vi "create report.vi"(8 "error in (no error)":errorcluster, 11 "TomoConversion in":refnum<class "TomoConversion.lvclass">) -> (0 "error out":errorcluster, 1 "correct number of subfolders":i32, 2 "Array":dbl[][](array[numeric]), 3 "TomoConversion out":refnum<class "TomoConversion.lvclass">)   [LabVIEW 2012, in "TomoConversion.lvclass"]
uses:
  TomoConversion.lvclass
  TomoConversion.lvclass/TomoConversion.ctl
  notice type.ctl
panel:
  out "j number y folders in this x 2":i32
  out "j number y folders in this x":i32
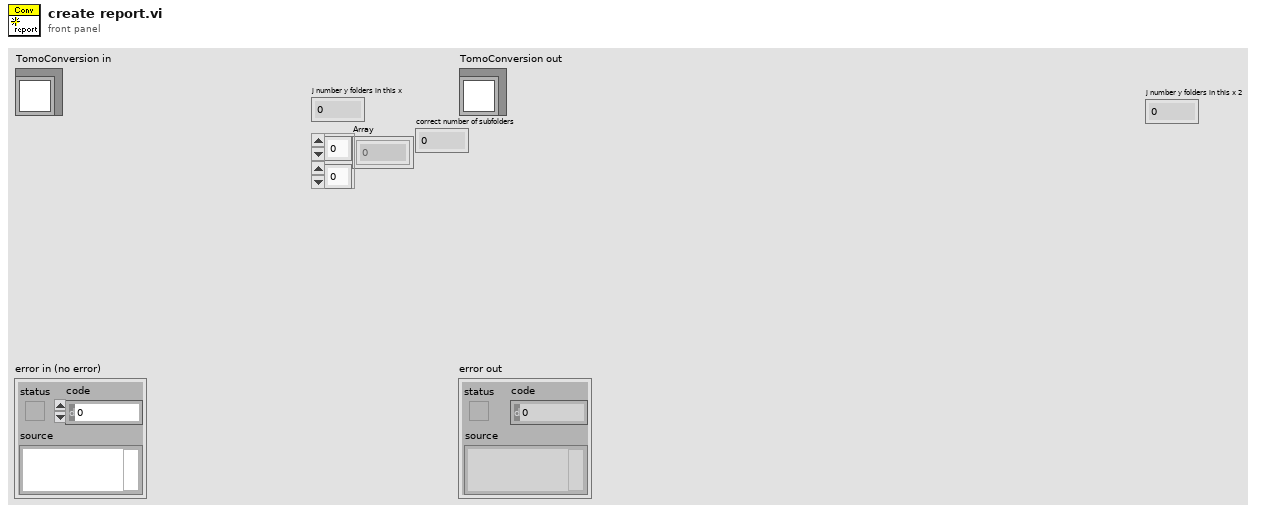
[diagram p1: front panel]
types:
  T1 = typedef "TomoConversion.lvclass/notice type.ctl" = enum16{"Grotto", "folder issue"}
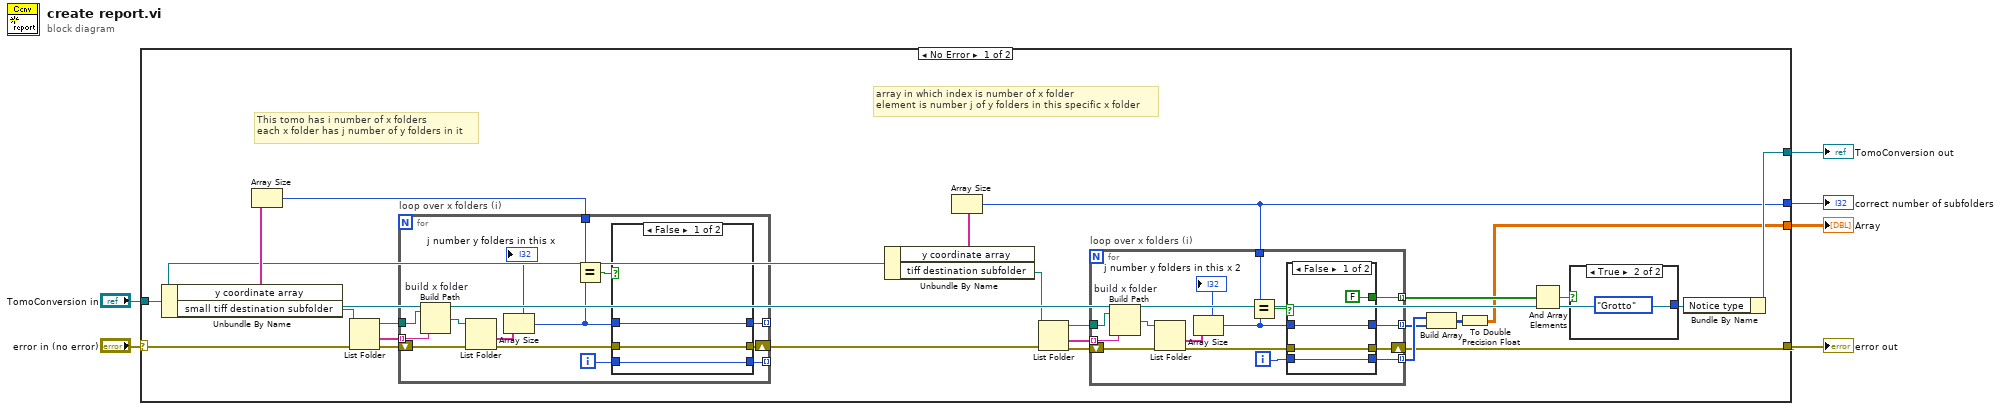
[diagram p0: block diagram]
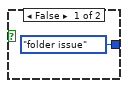
[diagram p2: hidden frame]
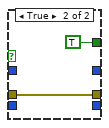
[diagram p3: hidden frame]
diagram:
  n1 = case shown="No Error" "error in (no error)" {
    selector: "error in (no error)" -> [w30 w71]
    tunnel: [w10 w71] -> w5
    tunnel: [w19 w70] -> w3
    tunnel: "TomoConversion in" -> [w20 w70]
    tunnel: [w8 _] -> w2
    tunnel: [w7 _] -> w1
    frame No Error {
      # "array in which index is number of x folder\nelement is number j of y folders in this specific x folder"
      # "This tomo has i number of x folders \neach x folder has j number of y folders in it"
      n2 = Unbundle By Name(w20) -> ("y coordinate array"=w26:string[], "small tiff destination subfolder"=w25:path)
      n3 = Array Size(array=w26) -> (size(s)=w16:i32)
      n4 = List Folder(path=w25, error in=w30) -> (path out=w27:path, folder names=w29:string[], error out=w28:errorcluster)  [unwired: 2 in, 1 out]
      n5 = for "loop over x folders (i)" {
        tunnel: w29 -> [w64] mode=indexing
        tunnel: w27 -> [w65]
        tunnel: [w54] -> _ mode=indexing
        shift-right: [w56] -> w15
        shift-left: w28 -> [w62]
        tunnel: w16 -> [w60]
        tunnel: [w53] -> _ mode=indexing
        i -> [w55]
        n6 = Build Path "build x folder"(base path=w65, name or relative path=w64) -> (appended path=w63:path)
        n7 = List Folder(path=w63, error in=w62) -> (folder names=w61:string[], error out=w57:errorcluster)  [unwired: 2 in, 2 out]
        n8 = Array Size(array=w61) -> (size(s)=w58:i32)
        "j number y folders in this x" <- w58
        n9 = Equal?(x=w60, y=w58) -> (x = y?=w59:bool)
        n10 = case shown="False" w59 {
          tunnel: w58 -> [w67 _]
          tunnel: [w67 _] -> w54
          tunnel: w57 -> [w68 w69]
          tunnel: [w68 w69] -> w56
          tunnel: w55 -> [w66 _]
          tunnel: [w66 _] -> w53
          frame False {
          }
          frame True {
            # "correct number of subfolders"
          }
        }
      }
      n11 = Unbundle By Name(w20) -> ("y coordinate array"=w24:string[], "tiff destination subfolder"=w11:path)
      n12 = Array Size(array=w24) -> (size(s)=w8:i32)
      n13 = List Folder(path=w11, error in=w15) -> (path out=w23:path, folder names=w21:string[], error out=w22:errorcluster)  [unwired: 2 in, 1 out]
      n14 = for "loop over x folders (i)" {
        tunnel: w21 -> [w45] mode=indexing
        tunnel: w23 -> [w46]
        tunnel: [w36] -> w12 mode=indexing
        shift-right: [w37] -> w10
        shift-left: w22 -> [w43]
        tunnel: w8 -> [w41]
        tunnel: [w34] -> w9 mode=indexing
        tunnel: [w33] -> w13 mode=indexing
        i -> [w35]
        n15 = Build Path "build x folder"(base path=w46, name or relative path=w45) -> (appended path=w44:path)
        n16 = List Folder(path=w44, error in=w43) -> (folder names=w42:string[], error out=w40:errorcluster)  [unwired: 2 in, 2 out]
        n17 = Array Size(array=w42) -> (size(s)=w38:i32)
        "j number y folders in this x 2" <- w38
        n18 = Equal?(x=w41, y=w38) -> (x = y?=w39:bool)
        n19 = case shown="False" w39 {
          tunnel: w40 -> [w50 w52]
          tunnel: w38 -> [w49 _]
          tunnel: [w50 w52] -> w37
          tunnel: [w49 _] -> w36
          tunnel: w35 -> [w48 _]
          tunnel: [w48 _] -> w33
          tunnel: [FALSE TRUE] -> w34
          frame False {
          }
          frame True {
          }
        }
      }
      n20 = Build Array(w13, w12) -> (w14:i32[][])
      n21 = To Double Precision Float(number=w14) -> (double precision float=w7:dbl[][])
      n22 = And Array Elements(Boolean array=w9) -> (logical AND=w18:bool)
      n23 = case shown="True" w18 {
        tunnel: [notice_type."folder issue" ("runtime.Notice type") notice_type."Grotto" ("runtime.Notice type")] -> w17
        frame False {
        }
        frame True {
        }
      }
      n24 = Bundle By Name(cluster=w20, "Notice type"=w17) -> (w19:refnum<class "TomoConversion.lvclass">)
    }
    frame Error {
    }
  }
  "error out" <- w5
  "TomoConversion out" <- w3
  "Array" <- w1
  "correct number of subfolders" <- w2
